vi "Enclose with Error Case Structure Core.vi"(8 "error in (no error)":errorcluster, 10 "block diagram in":refnum<vi>, 11 "VI in":refnum<vi>) -> (0 "error out":errorcluster, 2 "block diagram out":refnum<vi>, 3 "VI out":refnum<vi>)   [LabVIEW 2017]
uses:
  <vilib>/Utility/error.llb/Error Cluster From Error Code.vi
  <vilib>/ErrorRing/Error Ring.xnode
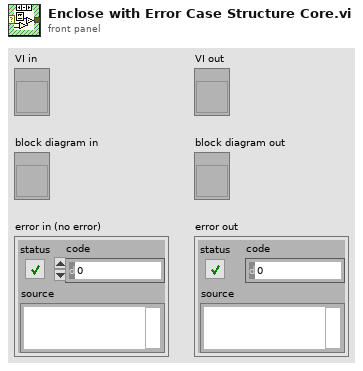
[diagram p1: front panel]
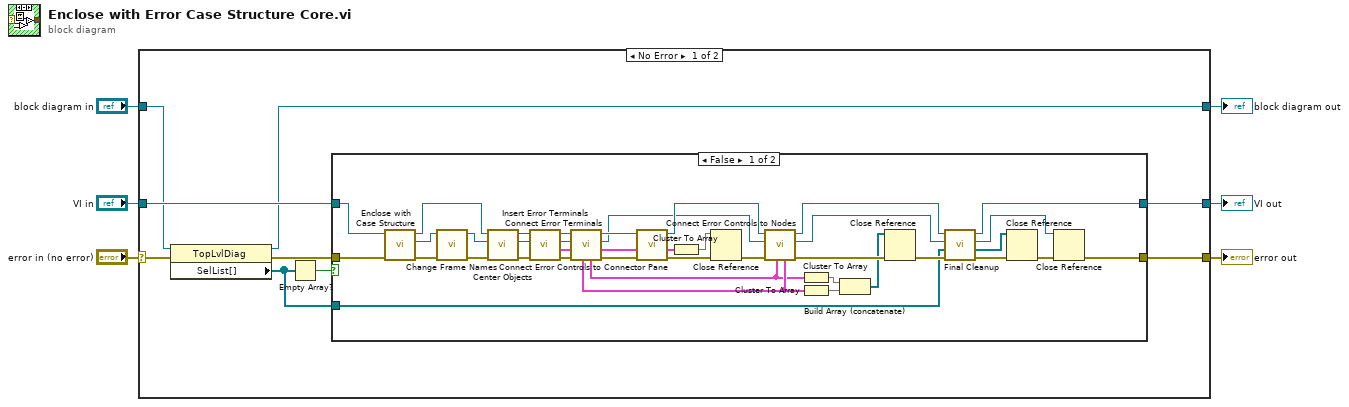
[diagram p0: block diagram]
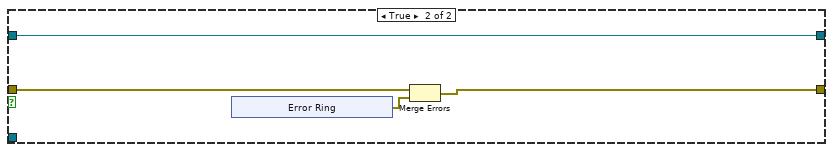
[diagram p2: hidden frame]
diagram:
  n1 = case shown="No Error" "error in (no error)" {
    selector: "error in (no error)" -> [w8 w66]
    tunnel: "VI in" -> [w14 w65]
    tunnel: "block diagram in" -> [w7 w64]
    tunnel: [w11 w64] -> w4
    tunnel: [w10 w65] -> w3
    tunnel: [w9 w66] -> w2
    frame No Error {
      n2 = property class="TopLvlDiag"(reference=w7, error in=w8) -> (reference out=w11:refnum<vi>, error out=w13:errorcluster, "SelList[]"=w15:refnum<vi>[])
      n3 = Empty Array?(array=w15) -> (empty?=w12:bool)
      n4 = case shown="False" w12 {
        tunnel: w13 -> [w52 w58]
        tunnel: w14 -> [w53 w56]
        tunnel: w15 -> [w29 _]
        tunnel: [w17 w56] -> w10
        tunnel: [w16 w57] -> w9
        frame False {
          n5 = call "Enclose with Case Structure.vi"("error in (no error)"=w52, "VI in"=w53) -> ("error out"=w51:errorcluster, "case structure"=w50:refnum<vi>, "VI out"=w47:refnum<vi>)  [unwired: 7 in]
          n6 = call "Change Frame Names.vi"("error in (no error)"=w51, "case structure in"=w50) -> ("error out"=w49:errorcluster, "case structure out"=w48:refnum<vi>)  [unwired: 8 in]
          n7 = call "Center Objects.vi"("error in (no error)"=w49, "case structure in"=w48, "VI in"=w47) -> ("error out"=w43:errorcluster, "case structure out"=w42:refnum<vi>, "VI out"=w46:refnum<vi>)  [unwired: 6 in]
          n8 = call "Insert Error Terminals.vi"("error in (no error)"=w43, "case structure in"=w42, "VI in"=w46) -> ("error out"=w45:errorcluster, "error controls"=w36:cluster{"in":refnum<vi>, "out":refnum<vi>}, "case structure out"=w35:refnum<vi>, "VI out"=w34:refnum<vi>)  [unwired: 5 in]
          n9 = call "Connect Error Terminals.vi"("error in (no error)"=w45, "error controls in"=w36, "case structure in"=w35, "VI in"=w34) -> ("error out"=w41:errorcluster, "error controls out"=w32:cluster{"in":refnum<vi>, "out":refnum<vi>}, "case structure out"=w19:refnum<vi>, "VI out"=w33:refnum<vi>, "error terminals"=w25:cluster{"in":refnum<vi>, "out":refnum<vi>}, "error case tunnels"=w26:cluster{"in":refnum<vi>, "out":refnum<vi>})  [unwired: 2 in]
          n10 = call "Connect Error Controls to Connector Pane.vi"("error in (no error)"=w41, "error controls in"=w32, "VI in"=w33) -> ("error out"=w40:errorcluster, "error controls out"=w31:cluster{"in":refnum<vi>, "out":refnum<vi>}, "VI out"=w21:refnum<vi>)  [unwired: 6 in]
          n11 = Cluster To Array(cluster=w31) -> (array=w30:refnum<vi>[])
          n12 = Close Reference(reference=w30, error in (no error)=w40) -> (error out=w37:errorcluster)
          n13 = call "Connect Error Controls to Nodes.vi"("error case tunnels in"=w26, "error terminals in"=w25, "error in (no error)"=w37, "case structure in"=w19, "VI in"=w21) -> ("error out"=w44:errorcluster, "case structure out"=w18:refnum<vi>, "VI out"=w20:refnum<vi>)  [unwired: 4 in]
          n14 = Cluster To Array(cluster=w25) -> (array=w23:refnum<vi>[])
          n15 = Cluster To Array(cluster=w26) -> (array=w24:refnum<vi>[])
          n16 = Build Array (concatenate)(w23, w24) -> (w22:refnum<vi>[])
          n17 = Close Reference(reference=w22, error in (no error)=w44) -> (error out=w54:errorcluster)
          n18 = call "Final Cleanup.vi"("error in (no error)"=w54, "initial selection list in"=w29, "case structure in"=w18, "VI in"=w20) -> ("error out"=w39:errorcluster, "initial selection list out"=w28:refnum<vi>[], "case structure out"=w27:refnum<vi>, "VI out"=w17:refnum<vi>)  [unwired: 4 in]
          n19 = Close Reference(reference=w28, error in (no error)=w39) -> (error out=w38:errorcluster)
          n20 = Close Reference(reference=w27, error in (no error)=w38) -> (error out=w16:errorcluster)
        }
        frame True {
          n21 = xnode "Error Ring"() -> ("error out"=w55:errorcluster)
          n22 = Merge Errors(w58, w55) -> (w57:errorcluster)
        }
      }
    }
    frame Error {
    }
  }
  "block diagram out" <- w4
  "VI out" <- w3
  "error out" <- w2
